vi "LeastDistanceAngle.vi"(4 "Sensor position":dbl, 5 "target angle (between pi and -pi)":dbl(knob) scale=3.14159..-3.14159) -> (0 "current angle (between pi and -pi)":dbl(knob) scale=3.14159..-3.14159, 1 "Reverse?":bool, 2 "motor output angle":dbl)   [LabVIEW 2014]
panel:
  out "within pi/2":dbl(knob) scale=3.14159..-3.14159
  out "straightforward delta":dbl(knob) scale=3.14159..-3.14159
  out "within pi":dbl(knob) scale=3.14159..-3.14159
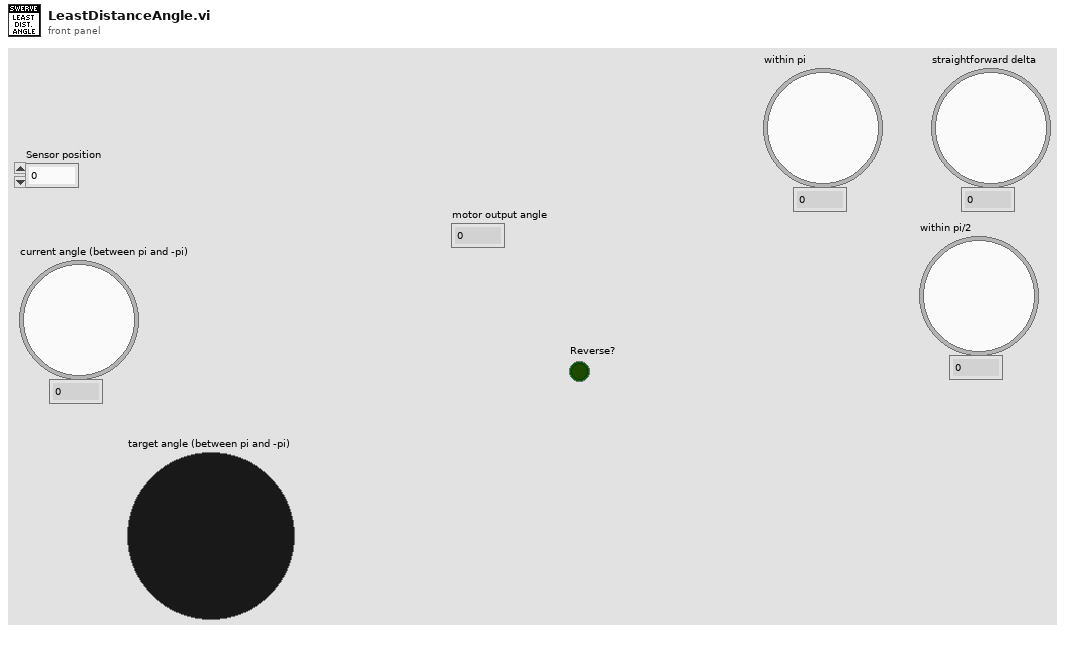
[diagram p1: front panel]
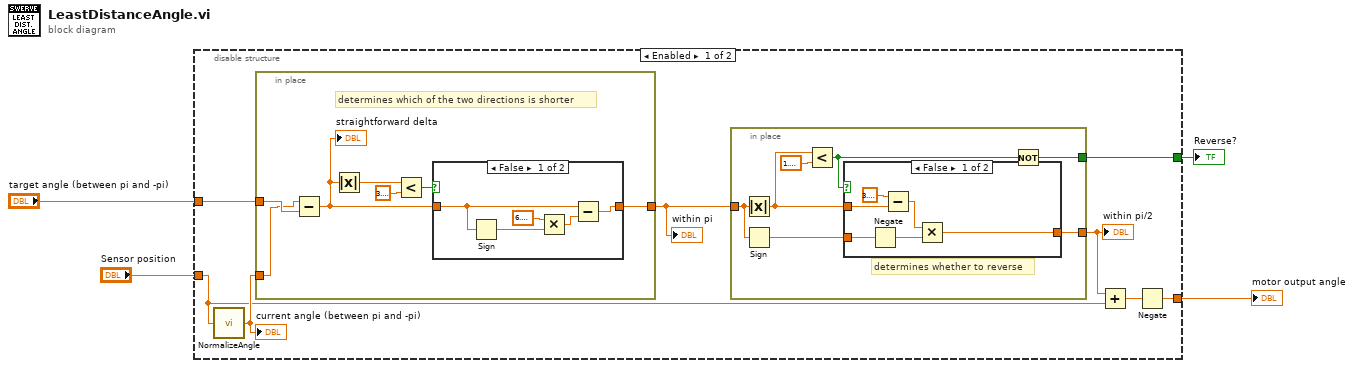
[diagram p0: block diagram]
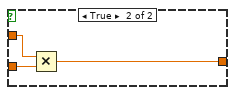
[diagram p2: hidden frame]
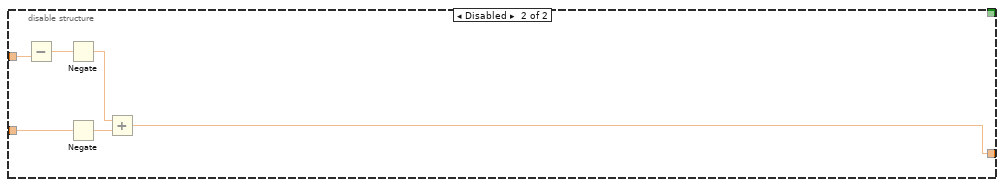
[diagram p4: hidden frame]
diagram:
  n1 = disable-structure shown="Enabled" {
    disable-tunnel: "target angle (between pi and -pi)" -> [w12 w45]
    disable-tunnel: [w11 _] -> w3
    disable-tunnel: "Sensor position" -> [w5 w44]
    disable-tunnel: [w7 w42] -> w1
    frame Enabled {
      n2 = call "NormalizeAngle.vi"("angle (rad)"=w5) -> ("angle (between pi and -pi)"=w8:dbl)
      "current angle (between pi and -pi)" <- w8
      n3 = in-place {
        in-place-border: w12 -> [w30]
        in-place-border: w8 -> [w29]
        in-place-border: [w31] -> w6
        # "determines which of the two directions is shorter"
        n4 = Subtract(x=w29, y=w30) -> (x-y=w35:dbl)
        "straightforward delta" <- w35
        n5 = Absolute Value(x=w35) -> (abs(x)=w34:dbl)
        n6 = Less?(x=w34, y=3.141592653589793) -> (x < y?=w33:bool)
        n7 = case shown="False" w33 {
          tunnel: w35 -> [w37 w41]
          tunnel: [w36 w41] -> w31
          frame False {
            n8 = Sign(1:w37) -> (0:w39:dbl)
            n9 = Multiply(x=6.283185307179586, y=w39) -> (x*y=w38:dbl)
            n10 = Subtract(x=w37, y=w38) -> (x-y=w36:dbl)
          }
          frame True {
          }
        }
      }
      "within pi" <- w6
      n11 = in-place {
        in-place-border: w6 -> [w19]
        in-place-border: [w15] -> w9
        in-place-border: [w13] -> w11
        # "determines whether to reverse"
        n12 = Absolute Value(x=w19) -> (abs(x)=w16:dbl)
        n13 = Sign(1:w19) -> (0:w17:dbl)
        n14 = Less?(x=w16, y=1.5707963267948966) -> (x < y?=w14:bool)
        n15 = case shown="False" w14 {
          tunnel: w17 -> [w22 w27]
          tunnel: w16 -> [w25 w28]
          tunnel: [w21 w26] -> w15
          frame False {
            n16 = Negate(x=w22) -> (-x=w20:dbl)
            n17 = Subtract(x=3.141592653589793, y=w25) -> (x-y=w23:dbl)
            n18 = Multiply(x=w23, y=w20) -> (x*y=w21:dbl)
          }
          frame True {
            n19 = Multiply(x=w28, y=w27) -> (x*y=w26:dbl)
          }
        }
        n20 = Not(x=w14) -> (.not. x?=w13:bool)
      }
      "within pi/2" <- w9
      n21 = Add(x=w9, y=w5) -> (x+y=w10:dbl)
      n22 = Negate(x=w10) -> (-x=w7:dbl)
    }
    frame Disabled {
      n23 = Subtract(y=w45) -> (x=w43:dbl, x-y=w48:dbl)
      n24 = Negate(x=w48) -> (-x=w47:dbl)
      n25 = Negate(x=w44) -> (-x=w46:dbl)
      n26 = Add(x=w47, y=w46) -> (x+y=w42:dbl)
    }
  }
  "motor output angle" <- w1
  "Reverse?" <- w3
